vi "Destructor.vi"(8 "error in (no error)":errorcluster, 11 "Singleton in":refnum<class "Provider.lvclass">) -> (0 "error out":errorcluster, 3 "Singleton out":refnum<class "Provider.lvclass">)   [LabVIEW 2020, in "Provider.lvlib" / "Provider.lvclass"]
uses:
  Provider.lvclass
  Provider.lvclass/Provider.ctl
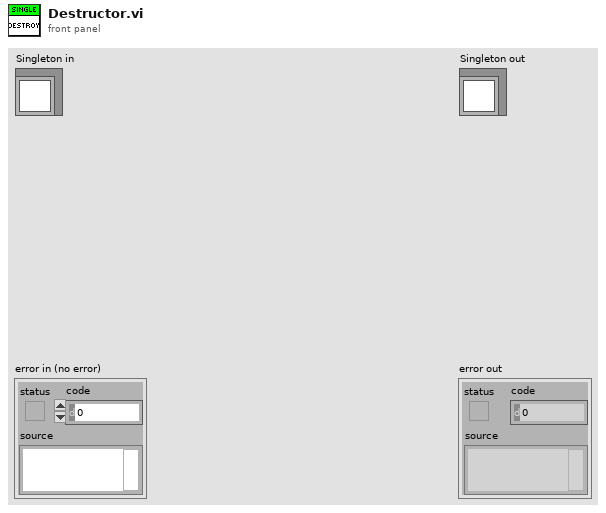
[diagram p1: front panel]
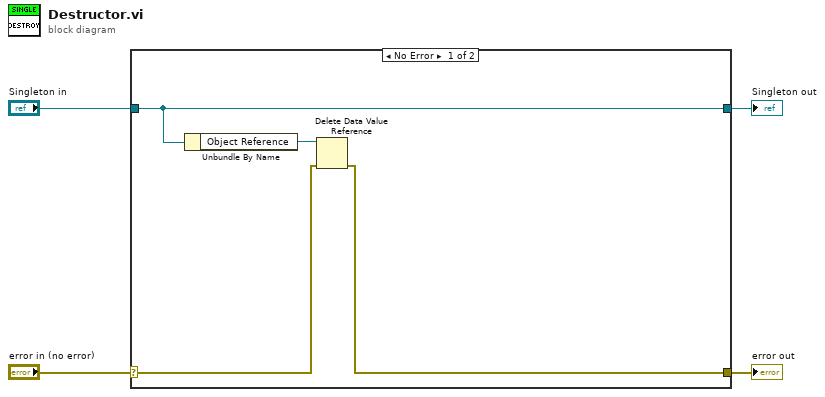
[diagram p0: block diagram]
diagram:
  n1 = case shown="No Error" "error in (no error)" {
    selector: "error in (no error)" -> [w6 w10]
    tunnel: [w5 w10] -> w3
    tunnel: [w8 w9] -> w1
    tunnel: "Singleton in" -> [w8 w9]
    frame No Error {
      n2 = Unbundle By Name(w8) -> ("Object Reference"=w7:refnum<data-value>)
      n3 = Delete Data Value Reference(data value reference=w7, error in=w6) -> (error out=w5:errorcluster)  [unwired: 1 out]
    }
    frame Error {
    }
  }
  "error out" <- w3
  "Singleton out" <- w1
